vi "Configure Waveform Modulation (AM).vi"(6 "AM Frequency (1000 Hz)":dbl=1000.0, 8 "error in (no error)":errorcluster, 9 "AM Depth Percentage (100)":i32=100, 10 "Waveform Generator Number (1: Waveform Generator 1)":i32(ring)=1 items=["Waveform Generator 1"=1], 11 "VISA resource name":refnum<visa-resource-name>) -> (0 "error out":errorcluster, 3 "VISA resource name out":refnum<visa-resource-name>)   [LabVIEW 2016, in "Agilent 2000 3000 X-Series.lvlib"]
doc: "Configures the waveform modulation AM."
uses:
  Agilent 2000 3000 X-Series.lvlib
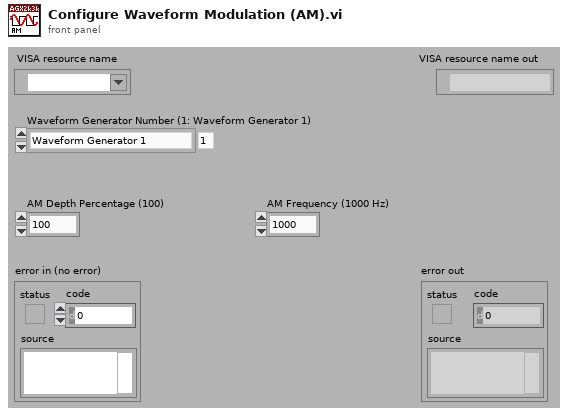
[diagram p1: front panel]
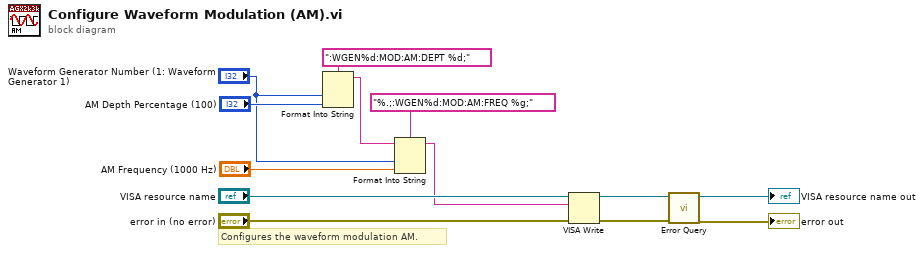
[diagram p0: block diagram]
diagram:
  # "Configures the waveform modulation AM."
  n1 = Format Into String(format string=":WGEN%d:MOD:AM:DEPT %d;", "Waveform Generator Number (1: Waveform Generator 1)", "AM Depth Percentage (100)") -> (resulting string=w5:string)  [unwired: 2 in, 1 out]
  n2 = Format Into String(format string="%.;:WGEN%d:MOD:AM:FREQ %g;", initial string=w5, "Waveform Generator Number (1: Waveform Generator 1)", "AM Frequency (1000 Hz)") -> (resulting string=w3:string)  [unwired: 1 in, 1 out]
  n3 = VISA Write(VISA resource name="VISA resource name", write buffer=w3, error in (no error)="error in (no error)") -> (VISA resource name out=w11:refnum<visa-resource-name>, error out=w10:errorcluster)  [unwired: 1 out]
  n4 = call "Error Query.vi"("error in (no error)"=w10, "VISA resource name"=w11) -> ("error out"=→"error out":errorcluster, "VISA resource name out"=→"VISA resource name out":refnum<visa-resource-name>)  [unwired: 8 out]
